vi "数值连接 (子VI).vi"(6 "DigNum引用句柄 4":refnum<vi>, 7 "x":i32, 9 "DigNum引用句柄 3":refnum<vi>, 10 "DigNum引用句柄输入":refnum<vi>, 11 "Digital输入":refnum<vi>) -> (3 "数据字符串":string)   [LabVIEW 2016]
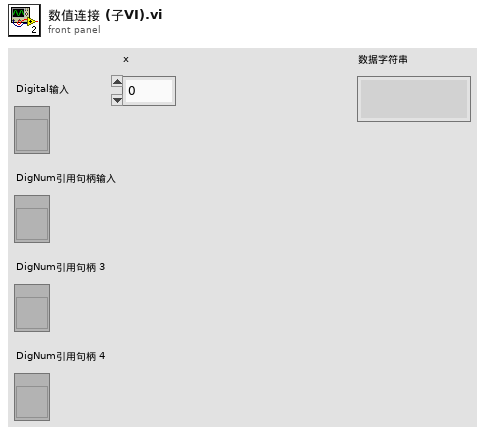
[diagram p1: front panel]
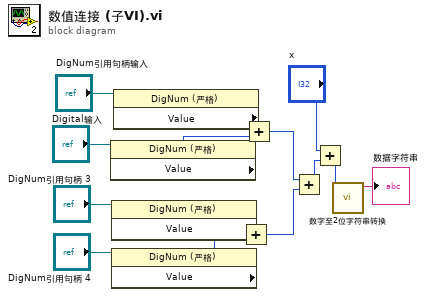
[diagram p0: block diagram]
diagram:
  n1 = property on="属性节点" class="DigNum (严格)"(reference="Digital输入") -> ("Value"=w10:i32)  [unwired: 1 in, 2 out]
  n2 = property on="属性节点" class="DigNum (严格)"(reference="DigNum引用句柄 3") -> ("Value"=w11:i32)  [unwired: 1 in, 2 out]
  n3 = property on="属性节点" class="DigNum (严格)"(reference="DigNum引用句柄 4") -> ("Value"=w12:i32)  [unwired: 1 in, 2 out]
  n4 = property on="属性节点" class="DigNum (严格)"(reference="DigNum引用句柄输入") -> ("Value"=w9:i32)  [unwired: 1 in, 2 out]
  n5 = Add(x=w11, y=w12) -> (x+y=w14:i32)
  n6 = Add(x=w9, y=w10) -> (x+y=w13:i32)
  n7 = Add(x=w13, y=w14) -> (x+y=w3:i32)
  n8 = Add(x="x", y=w3) -> (x+y=w1:i32)
  n9 = call "数字至2位字符串转换.vi"("数值"=w1) -> ("数据字符串"=→"数据字符串":string)  [unwired: 10 in]
